vi "RS232C-Dialog.vi"() -> (0 "cancelled":bool, 1 "VISA resource name":refnum<visa-resource-name>="COM1")   [LabVIEW 2013]
panel:
  in  "cancel":bool
  in  "select":bool
  in  "Please select serial interface ...":i32(listbox)
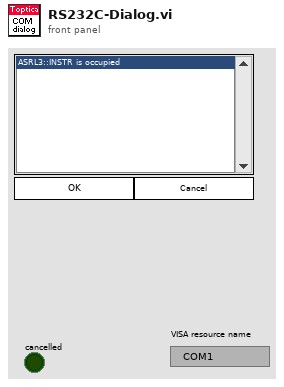
[diagram p1: front panel]
types:
  T1 = cluster{"friendlyName":string, "VISAname":string}[]
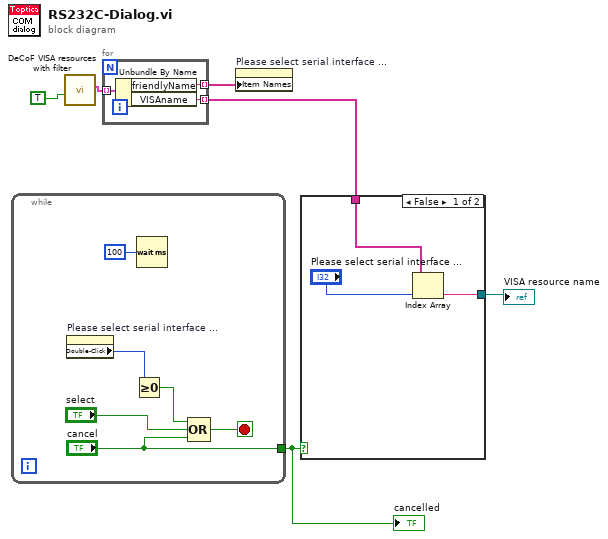
[diagram p0: block diagram]
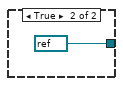
[diagram p2: hidden frame]
diagram:
  n1 = while {
    tunnel: ["cancel"] -> w3
    stop <- w9 stop-if-true
    n2 = property on="Please select serial interface ..." class="LstBox (strict)"() -> ("Double-Click"=w12:i32)  [unwired: 2 in, 2 out]
    n3 = Greater Or Equal To 0?(x=w12) -> (x >= 0?=w10:bool)
    n4 = Wait (ms)(milliseconds to wait=u32 100) -> ()  [unwired: 1 out]
    n5 = Compound Arithmetic op=OR(w10, "select", "cancel") -> (w9:bool)
  }
  "cancelled" <- w3
  n6 = call "DeCoF VISA resources with filter.vi"("apply filter"=TRUE) -> ("Array"=w5:T1)  [unwired: 5 in, 1 out]
  n7 = for {
    tunnel: w5 -> [w15] mode=indexing
    tunnel: [w14] -> w4 mode=indexing
    tunnel: [w13] -> w2 mode=indexing
    n8 = Unbundle By Name(w15) -> ("friendlyName"=w14:string, "VISAname"=w13:string)
  }
  n9 = property on="Please select serial interface ..." class="LstBox (strict)"("Item Names"=w4) -> ()  [unwired: 2 in, 2 out]
  n10 = case shown="False" w3 {
    tunnel: w2 -> [w18 _]
    tunnel: [w16 refnum<visa-resource-name> refnum ("VISA resource name")] -> w1
    frame False {
      n11 = Index Array(array=w18, index="Please select serial interface ...") -> (element=w16:string)
    }
    frame True {
    }
  }
  "VISA resource name" <- w1
